vi "RankCompare.vi"(8 "error in (no error)":errorcluster, 10 "Threshold":T1=enum."INFO", 11 "Level":T1=enum."INFO") -> (0 "error out":errorcluster, 3 "Passes":bool)   [LabVIEW 2026, in "Lumberjack.lvlib"]
doc: "Pure severity comparison for threshold gating. Returns TRUE when Level passes Threshold, i.e. rank(Level) <= rank(Threshold), using the Severity enum ordinal as the rank (SRS-LMBR-005, 006). Used on the hot path by Log (stage-1) and by HandleStatement (stage-2). No state, no I/O; deterministic and unit-testable."
uses:
  Lumberjack.lvlib
  TypeDefs/Severity.ctl
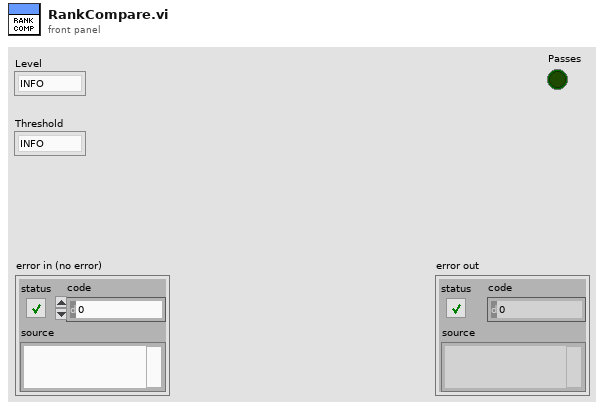
[diagram p1: front panel]
types:
  T1 = typedef "Lumberjack.lvlib/Severity.ctl" = enum16{"OFF", "FATAL", "ERROR", "WARN", "INFO", "DEBUG", "TRACE", "ALL"}
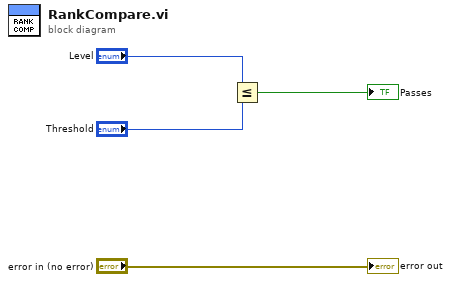
[diagram p0: block diagram]
diagram:
  n1 = Less Or Equal?(x="Level", y="Threshold") -> (x <= y?=→"Passes":bool)
  "error out" <- "error in (no error)"
